vi "Initialize.vi"(0 "Hotel Management Tool Model in":refnum<class "Hotel Management Tool Model.lvclass">, 11 "error in (no error)":errorcluster) -> (4 "Hotel Management Tool Model out":refnum<class "Hotel Management Tool Model.lvclass">, 15 "error out":errorcluster)   [LabVIEW 2023, in "Hotel Management Tool Model.lvlib" / "Hotel Management Tool Model.lvclass"]
uses:
  Hotel Management Tool Model.lvclass
  C:/Program Files/National Instruments/LabVIEW 2023/vi.lib/ActorFramework/Actor/Actor.lvclass
  Hotel Management Tool UI/Hotel Management Tool UI/Hotel Management Tool UI.lvclass
  Hotel Management Tool Model Messages/Launch Rooms Manager Msg/Launch Rooms Manager Msg.lvclass
  C:/Users/bhaghyaraj/Trainings/NI Actor Framework/SDLC/Hotel Management Tool UI/Hotel Management Tool UI Messages/Launch Rooms Manager Msg/Launch Rooms Manager Msg.lvclass
  Hotel Management Tool UI/Hotel Management Tool UI/Hotel Management Tool UI.lvclass/Hotel Management Tool UI.ctl
  Hotel Management Tool Model.lvclass/Hotel Management Tool Model.ctl
  <vilib>/ActorFramework/Actor/Actor.lvclass/Actor.ctl
  <vilib>/ActorFramework/Message Enqueuer/Message Enqueuer.lvclass/Message Enqueuer.ctl
  <vilib>/ActorFramework/Message Enqueuer/Init from Existing Queue.vi
  <vilib>/ActorFramework/Message Enqueuer/Enqueue.vi
  Hotel Management Tool Model Messages/Launch Database Msg/Launch Database Msg.lvclass
  C:/Program Files/National Instruments/LabVIEW 2023/vi.lib/ActorFramework/Message/Message.lvclass
  Hotel Management Tool Model Messages/Launch Restaurant Manager Msg/Launch Restaurant Manager Msg.lvclass
  Hotel Management Tool Model Messages/Launch Staff Manager Msg/Launch Staff Manager Msg.lvclass
  <vilib>/ActorFramework/Message Priority Queue/Priority Enqueue.vi
  <vilib>/ActorFramework/Message Enqueuer/Message Enqueuer.lvclass
  <vilib>/ActorFramework/Actor/Actor.lvclass
  Hotel Management Tool Model Messages/Launch Room Service Monitor Msg/Launch Room Service Monitor Msg.lvclass
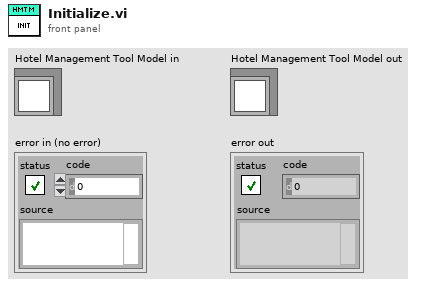
[diagram p1: front panel]
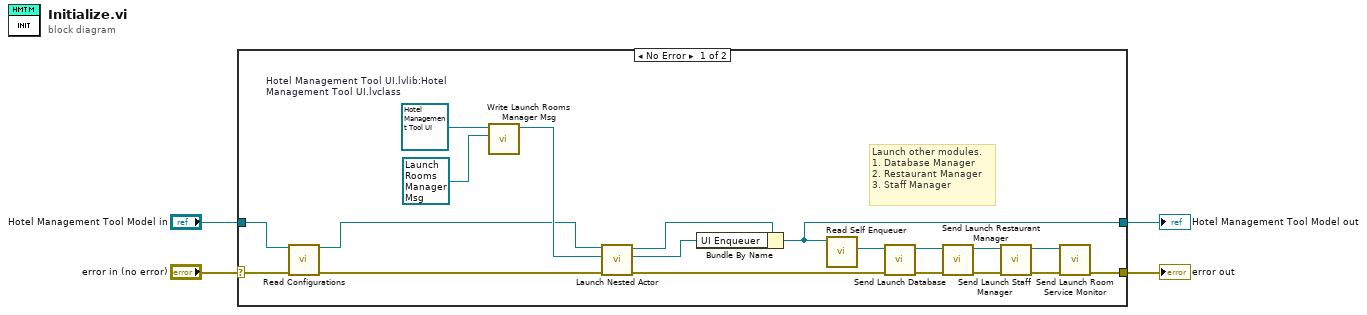
[diagram p0: block diagram]
diagram:
  n1 = case shown="No Error" "error in (no error)" {
    selector: "error in (no error)" -> [w19 w25]
    tunnel: [w6 w25] -> w3
    tunnel: [w14 w24] -> w1
    tunnel: "Hotel Management Tool Model in" -> [w16 w24]
    frame No Error {
      w21 = refnum<class "Hotel Management Tool UI.lvclass"> refnum  # Hotel Management Tool UI.lvlib:Hotel Management Tool UI.lvclass
      # "Launch other modules.\n1. Database Manager\n2. Restaurant Manager\n3. Staff Manager"
      n2 = call "Read Configurations.vi"("Hotel Management Tool Model in"=w16, "error in (no error)"=w19) -> ("Hotel Management Tool Model out"=w15:refnum<class "Hotel Management Tool Model.lvclass">, "error out"=w17:errorcluster)  [unwired: 12 in]
      n3 = call "Write Launch Rooms Manager Msg.vi"("Hotel Management Tool UI.lvlib:Launch Rooms Manager Msg.lvclass"=refnum<class "Launch Rooms Manager Msg.lvclass"> refnum ("Hotel Management Tool Model.lvlib:Launch Rooms Manager Msg.lvclass"), "Hotel Management Tool UI in"=w21) -> ("Hotel Management Tool UI out"=w20:refnum<class "Hotel Management Tool UI.lvclass">)  [unwired: 9 in]
      n4 = call <vilib>:"Launch Nested Actor.vi"("error in (no error)"=w17, "Nested Actor"=w20, "Caller Actor in"=w15) -> ("error out"=w9:errorcluster, "Nested Actor's Enqueuer"=w22:refnum<class "Message Enqueuer.lvclass">, "Caller Actor out"=w23:refnum<class "Hotel Management Tool Model.lvclass">)  [unwired: 6 in]
      n5 = Bundle By Name(cluster=w23, "UI Enqueuer"=w22) -> (w14:refnum<class "Hotel Management Tool Model.lvclass">)
      n6 = call <vilib>:"Read Self Enqueuer.vi"("Actor"=w14) -> ("Self Enqueuer"=w7:refnum<class "Message Enqueuer.lvclass">)  [unwired: 10 in]
      n7 = call "Send Launch Database.vi"("error in (no error)"=w9, "Message Enqueuer"=w7) -> ("error out"=w12:errorcluster, "Message Enqueuer out"=w13:refnum<class "Message Enqueuer.lvclass">)  [unwired: 8 in]
      n8 = call "Send Launch Restaurant Manager.vi"("error in (no error)"=w12, "Message Enqueuer"=w13) -> ("error out"=w10:errorcluster, "Message Enqueuer out"=w11:refnum<class "Message Enqueuer.lvclass">)  [unwired: 8 in]
      n9 = call "Send Launch Staff Manager.vi"("error in (no error)"=w10, "Message Enqueuer"=w11) -> ("error out"=w8:errorcluster, "Message Enqueuer out"=w5:refnum<class "Message Enqueuer.lvclass">)  [unwired: 8 in]
      n10 = call "Send Launch Room Service Monitor.vi"("error in (no error)"=w8, "Message Enqueuer"=w5) -> ("error out"=w6:errorcluster)  [unwired: 8 in, 1 out]
    }
    frame Error {
    }
  }
  "error out" <- w3
  "Hotel Management Tool Model out" <- w1
